vi "Untitled 6 (SubVI).vi"(6 "Numeric in":i32, 9 "Numeric 4":i32, 10 "Numeric 3":i32, 11 "Numeric 5":i32) -> (0 "y":i32, 1 "x":i32, 3 "Numeric out":dbl)   [LabVIEW 2014]
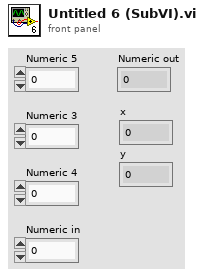
[diagram p1: front panel]
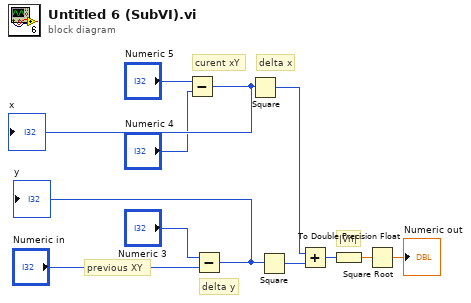
[diagram p0: block diagram]
diagram:
  # "delta y"
  # "delta x"
  # "|Vn|"
  # "previous XY"
  # "curent xY"
  n1 = Subtract(x="Numeric 5", y="Numeric 4") -> (x-y=w7:i32)
  "x" <- w7
  n2 = Subtract(x="Numeric 3", y="Numeric in") -> (x-y=w8:i32)
  "y" <- w8
  n3 = Square(x=w7) -> (x^2=w9:i32)
  n4 = Square(x=w8) -> (x^2=w10:i32)
  n5 = Add(x=w9, y=w10) -> (x+y=w11:i32)
  n6 = To Double Precision Float(number=w11) -> (double precision float=w2:dbl)
  n7 = Square Root(x=w2) -> (sqrt(x)=→"Numeric out":dbl)
